vi "DAQ- Steper.vi"(0 "Travel (Degree)":dbl=100.0, 1 "Mode":i32(ring)=10178 items=["Finite Samples"=10178, "Continuous Samples"=10123, "Hardware Timed Single Point"=12522], 5 "Home Condition":bool, 7 "Speed d/s":dbl=10.0, 11 "error in":errorcluster) -> (4 "Task Done Bit":bool, 14 "error out":errorcluster)   [LabVIEW 2015]
uses:
  Project Setup/Globle Variable/GR_Servo.vi
  Galobal variable_TI.vi
  <vilib>/DAQmx/create/channels.llb/DAQmx Create Channel (CO-Pulse Generation-Frequency).vi
  <vilib>/DAQmx/configure/timing.llb/DAQmx Timing (Implicit).vi
panel:
  in  "Motor PPR":dbl=3600.0
  in  "Motor Gear Ratio":dbl=1.0
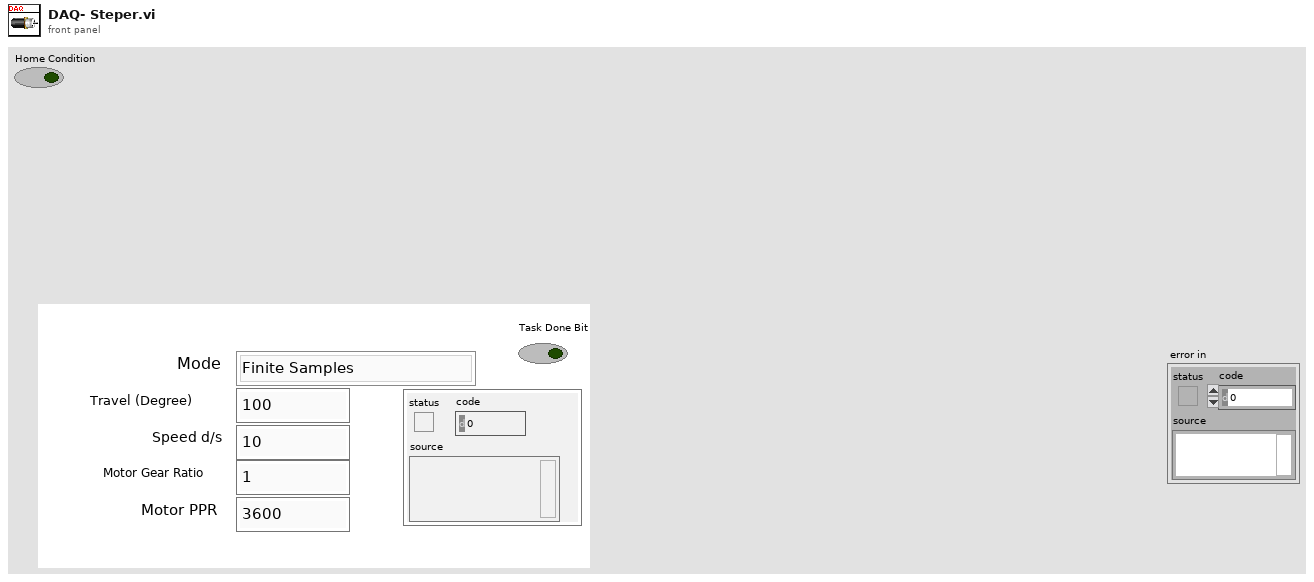
[diagram p1: front panel]
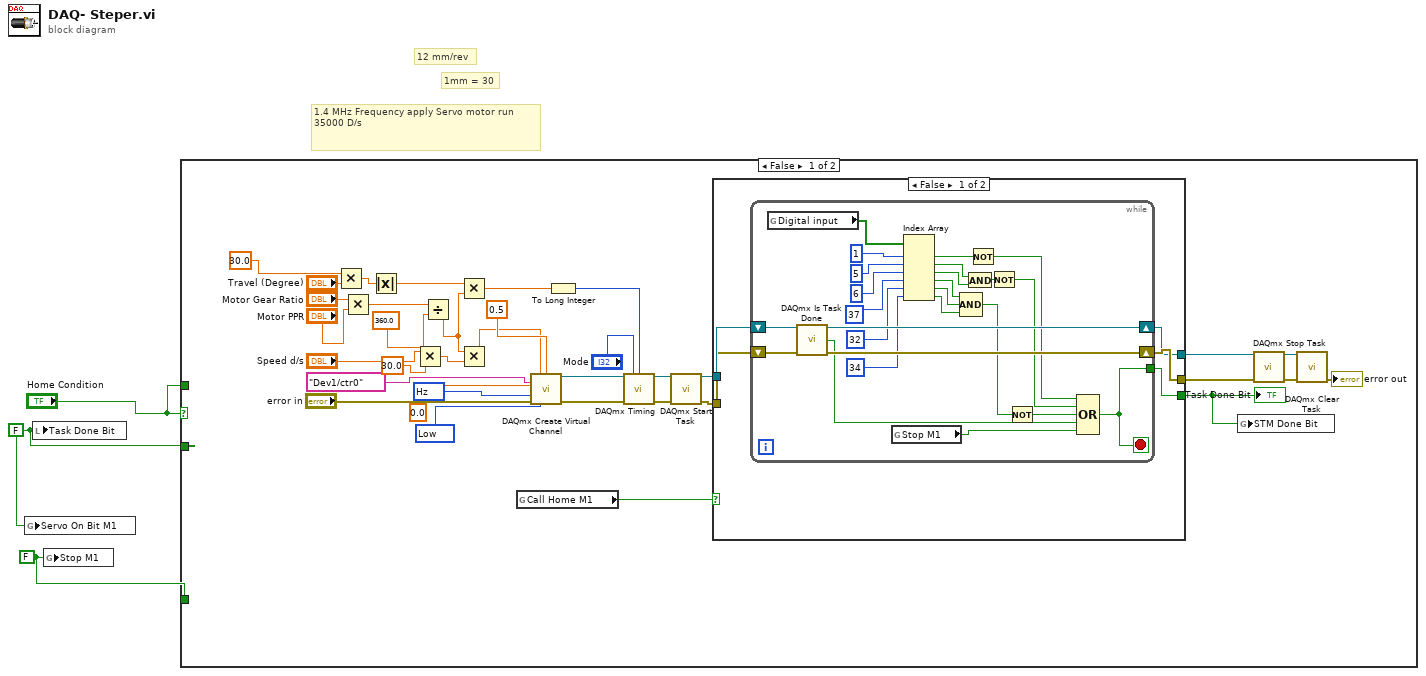
[diagram p0: block diagram]
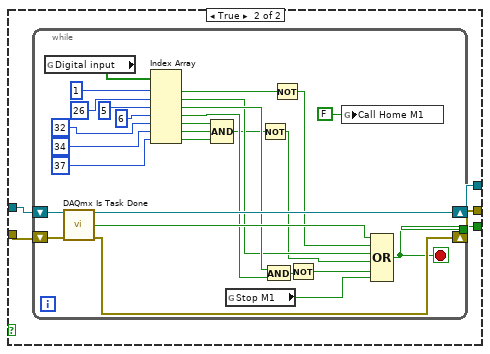
[diagram p2: hidden frame]
diagram:
  w2 = FALSE ("Stop M1")
  w3 = FALSE ("Task Done Bit")
  # "1mm = 30"
  # "12 mm/rev"
  # "1.4 MHz Frequency apply Servo motor run \n35000 D/s"
  n1 = global write "GR_Servo.vi" "Servo On Bit M1"(w3) -> ()
  n2 = local write "Task Done Bit"(w3) -> ()
  n3 = global write "Galobal variable_TI.vi" "Stop M1"(w2) -> ()
  n4 = case shown="False" "Home Condition" {
    tunnel: w3 -> [_ _]
    tunnel: w2 -> [_ _]
    tunnel: "Home Condition" -> [_ _]
    frame False {
      w14 = 10373 items=["Hz"=10373] ("units")
      w15 = 10214 items=["High"=10192, "Low"=10214] ("idle state")
      n5 = Multiply(x=30.0, y="Travel (Degree)") -> (x*y=w10:dbl)
      n6 = Multiply(x="Motor Gear Ratio", y="Motor PPR") -> (x*y=w24:dbl)
      n7 = Absolute Value(x=w10) -> (abs(x)=w23:dbl)
      n8 = Multiply(x="Speed d/s", y=30.0) -> (x*y=w8:dbl)
      n9 = Divide(x=w24, y=360.0) -> (x/y=w30:dbl)
      n10 = Multiply(x=w23, y=w30) -> (x*y=w28:dbl)
      n11 = Multiply(x=w30, y=w8) -> (x*y=w35:dbl)
      n12 = global read "Galobal variable_TI.vi" "Call Home M1"() -> (w5:bool)
      n13 = call-poly <vilib>:"DAQmx Create Virtual Channel.vi"("frequency"=w35, "duty cycle"=0.5, "counter"=tag "Dev1/ctr0", "units"=w14, "error in"="error in", "idle state"=w15, "initial delay"=0.0) -> ("task out"=w17:refnum<k21>, "error out"=w18:errorcluster)  [unwired: 7 in]
      n14 = To Long Integer(number=w28) -> (32bit integer=w38:i32)
      n15 = call-poly <vilib>:"DAQmx Timing.vi"("task/channels in"=w17, "sample mode"="Mode", "samples per channel"=w38, "error in"=w18) -> ("task out"=w19:refnum<k21>, "error out"=w20:errorcluster)  [unwired: 10 in]
      n16 = call <vilib>:"DAQmx Start Task.vi"("task/channels in"=w19, "error in"=w20) -> ("task out"=w13:refnum<k21>, "error out"=w11:errorcluster)  [unwired: 12 in]
      n17 = case shown="False" w5 {
        tunnel: [w43 w70] -> w33
        tunnel: w13 -> [w42 w73]
        tunnel: [w41 w71] -> w12
        tunnel: w11 -> [w40 w72]
        tunnel: [w39 w69] -> w4
        frame False {
          n18 = while {
            shift-right: [w66] -> w41
            shift-left: w42 -> [w68]
            shift-right: [w67] -> w43
            shift-left: w40 -> [w65]
            tunnel: [w64] -> w39
            stop <- w64 stop-if-true
            n19 = global read "Galobal variable_TI.vi" "Digital input"() -> (w63:bool[])
            n20 = call <vilib>:"DAQmx Is Task Done.vi"("task/channels in"=w68, "error in"=w65) -> ("task out"=w66:refnum<k21>, "task done?"=w60:bool, "error out"=w67:errorcluster)  [unwired: 11 in]
            n21 = global read "Galobal variable_TI.vi" "Stop M1"() -> (w61:bool)
            n22 = Index Array(array=w63, index #1=1 ("index"), index #2=5 ("index"), index #3=6 ("index"), index #4=37 ("index"), index #5=32 ("index"), index #6=34 ("index")) -> (element #1=w59:bool, element #2=w56:bool, element #3=w55:bool, element #4=w50:bool, element #5=w49:bool, element #6=w48:bool)
            n23 = Compound Arithmetic op=AND(w50, w49, w48) -> (w45:bool)
            n24 = And(x=w56, y=w55) -> (x .and. y?=w54:bool)
            n25 = Not(x=w59) -> (.not. x?=w47:bool)
            n26 = Not(x=w54) -> (.not. x?=w46:bool)
            n27 = Not(x=w45) -> (.not. x?=w44:bool)
            n28 = Compound Arithmetic op=OR(w47, w46, w44, w60, w61) -> (w64:bool)
          }
        }
        frame True {
          n29 = while {
            shift-right: [w99] -> w71
            shift-left: w73 -> [w101]
            shift-right: [w100] -> w70
            shift-left: w72 -> [w98]
            tunnel: [w95] -> w69
            stop <- w95 stop-if-true
            n30 = global read "Galobal variable_TI.vi" "Digital input"() -> (w96:bool[])
            n31 = call <vilib>:"DAQmx Is Task Done.vi"("task/channels in"=w101, "error in"=w98) -> ("task out"=w99:refnum<k21>, "task done?"=w92:bool, "error out"=w100:errorcluster)  [unwired: 11 in]
            n32 = Index Array(array=w96, index #1=1 ("index"), index #2=26 ("index"), index #3=5 ("index"), index #4=6 ("index"), index #5=32 ("index"), index #6=34 ("index"), index #7=37 ("index")) -> (element #1=w91:bool, element #2=w85:bool, element #3=w88:bool, element #4=w87:bool, element #5=w79:bool, element #6=w78:bool, element #7=w77:bool)
            n33 = Compound Arithmetic op=AND(w79, w78, w77) -> (w75:bool)
            n34 = global read "Galobal variable_TI.vi" "Stop M1"() -> (w76:bool)
            n35 = Not(x=w75) -> (.not. x?=w74:bool)
            n36 = And(x=w88, y=w87) -> (x .and. y?=w86:bool)
            n37 = Not(x=w91) -> (.not. x?=w83:bool)
            n38 = Not(x=w86) -> (.not. x?=w84:bool)
            n39 = global write "Galobal variable_TI.vi" "Call Home M1"(FALSE ("Call Home M1")) -> ()
            n40 = Compound Arithmetic op=OR(w92, w83, w85, w74, w84, w76) -> (w95:bool)
          }
        }
      }
      "Task Done Bit" <- w4
      n41 = global write "Galobal variable_TI.vi" "STM Done Bit"(w4) -> ()
      n42 = call <vilib>:"DAQmx Stop Task.vi"("task/channels in"=w12, "error in"=w33) -> ("task out"=w21:refnum<k21>, "error out"=w34:errorcluster)  [unwired: 12 in]
      n43 = call <vilib>:"DAQmx Clear Task.vi"("task in"=w21, "error in"=w34) -> ("error out"=→"error out":errorcluster)  [unwired: 13 in]
    }
    frame True {
    }
  }
